vi "Register.vi"(6 "picture":refnum<vi>) -> (0 "error out":errorcluster)   [LabVIEW 2013]
uses:
  ROS/Code/SubVIs/BaxterSide.ctl
  ROS/Code/Console/Servers/ServerSubs/(nist) Arm Globals.vi
  <vilib>/Utility/config.llb/Read Key (String).vi
  <vilib>/Utility/config.llb/Read Key (Double).vi
  <vilib>/Utility/config.llb/Write Key (String).vi
  <vilib>/Utility/config.llb/NI_LVConfig.lvlib
panel:
  in  "Side":T1=enum."right"
  in  "Object":string
  in  "Tab Control":T2(tab)=enum."Calibration Table"
  out "picture 2":picture
  out "Progress":T3
  out "Table":dbl[][](array[numeric]) caption="FL\nFR\nNL\nNR" format="%.1f"
  # "Basic Commands are:\n   Convert   - convert offset to joints\n   Current   - current joint and offset\n   Register  - determine position\n   Save      - save calibration data\n   Load      - load calibration data\n   Reference - give reference joint position"
  # "Position gripper over center before starting"
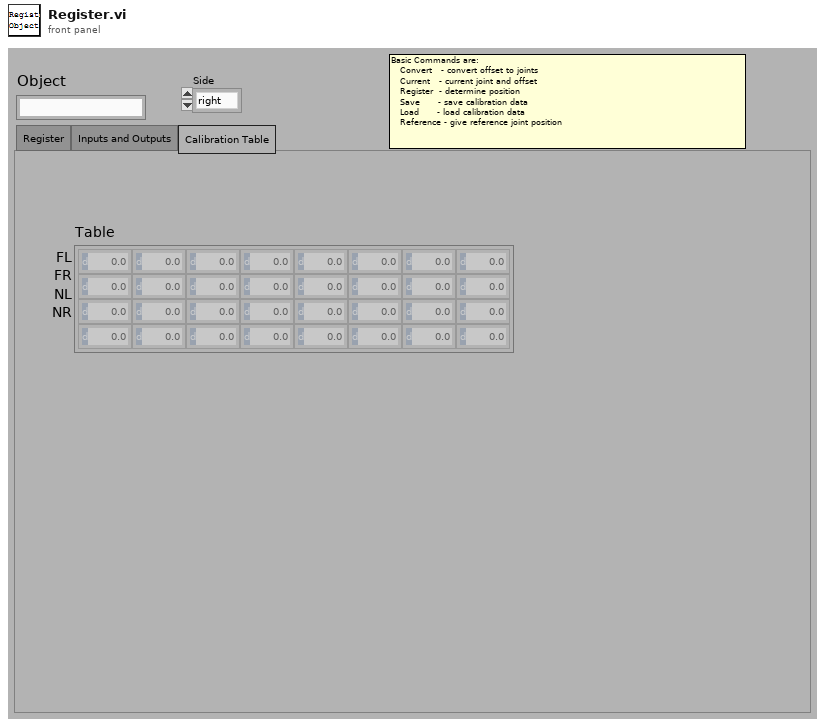
[diagram p1: front panel]
types:
  T1 = typedef "BaxterSide.ctl" = enum16{"left", "right"}
  T2 = enum32{"Register", "Inputs and Outputs", "Calibration Table"}
  T3 = cluster{"FL":bool, "FR":bool, "NL":bool, "NR":bool}
  T4 = cluster{"X":dbl, "Y":dbl, "Z":dbl, "O":dbl, "A":dbl, "T":dbl}
  T5 = typedef "NI_LVConfig.lvlib/Config Data RefNum.ctl" = refnum<k1>
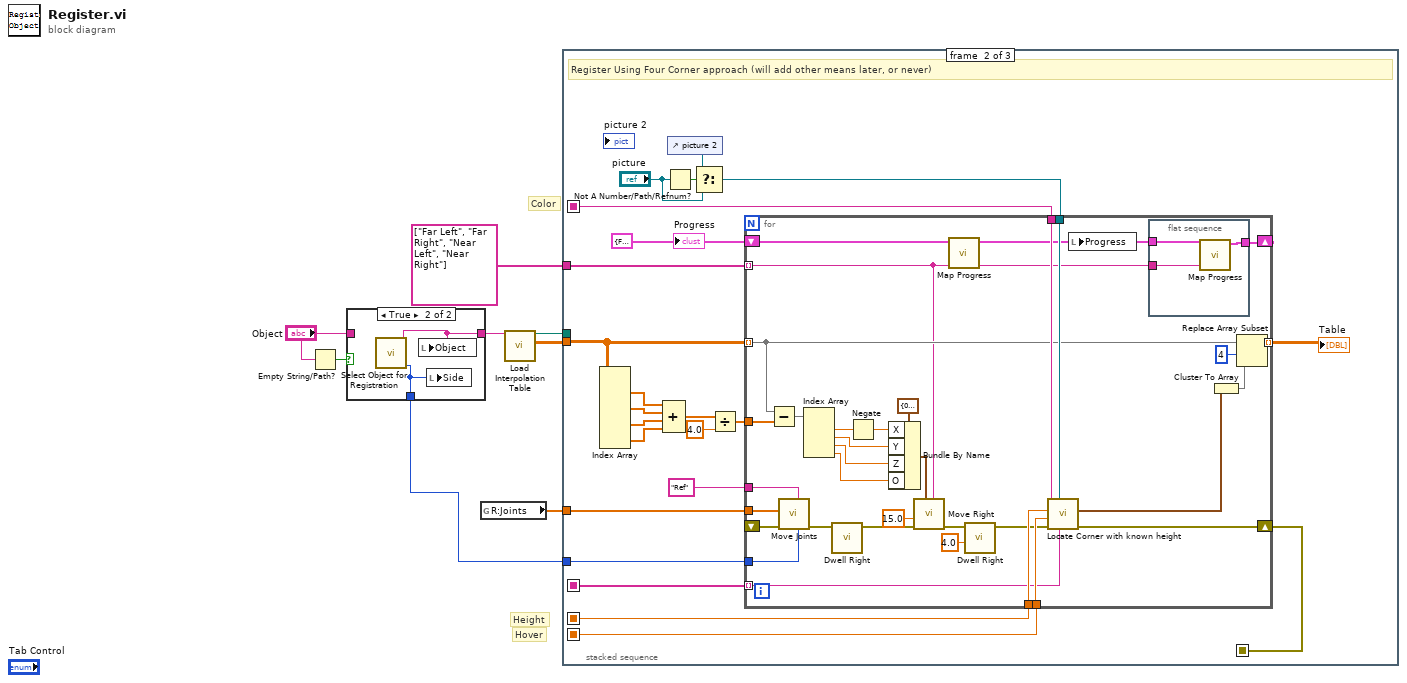
[diagram p0: block diagram]
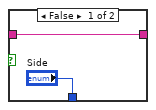
[diagram p2: hidden frame]
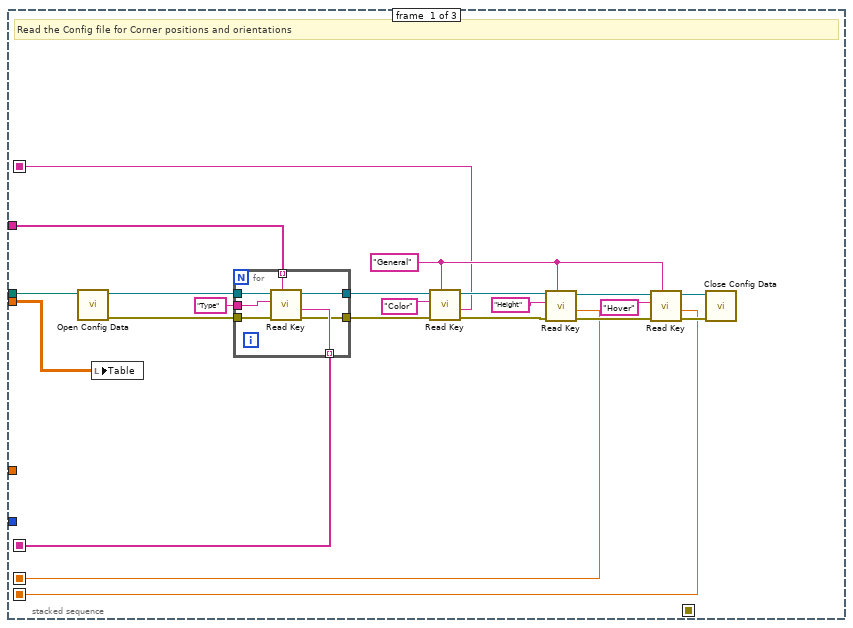
[diagram p3: hidden frame]
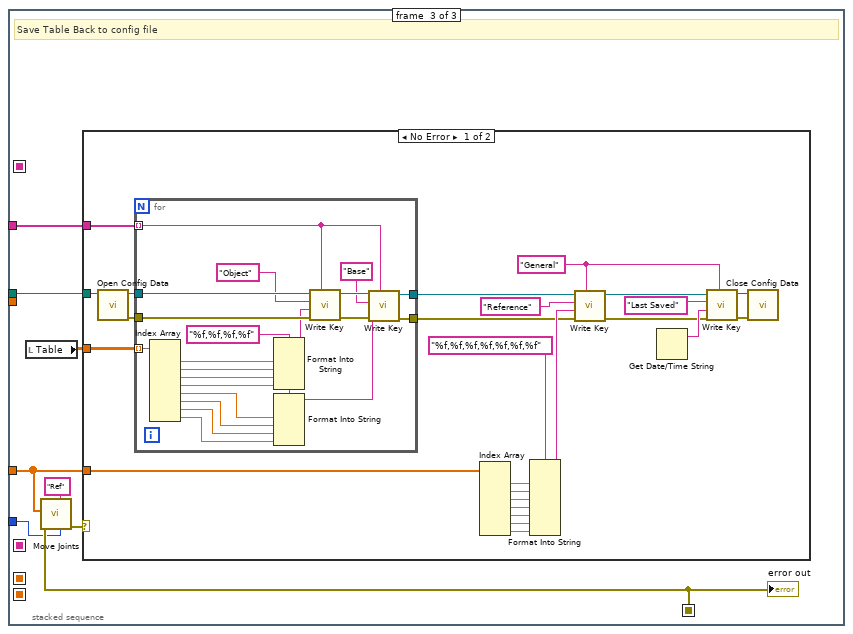
[diagram p4: hidden frame]
diagram:
  # "Color"
  # "Hover"
  # "Height"
  n1 = Empty String/Path?(string/path="Object") -> (empty?=w6:bool)
  n2 = case shown="True" w6 {
    tunnel: "Object" -> [w9 _]
    tunnel: ["Side" w11] -> w4
    tunnel: [w9 w12] -> w1
    frame False {
    }
    frame True {
      n3 = call "Select Object for Registration.vi"() -> ("Side"=w11:T1, "Object"=w12:string)  [unwired: 9 in, 1 out]
      n4 = local write "Object"(w12) -> ()
      n5 = local write "Side"(w11) -> ()
    }
  }
  n6 = global read "(nist) Arm Globals.vi" "R:Joints"() -> (w8:dbl[])
  n7 = call "Load Interpolation Table.vi"("Object Name"=w1) -> ("Table"=w3:dbl[][], "File"=w2:path)  [unwired: 7 in, 2 out]
  n8 = stacked-sequence {
    seq-local: [w15 _ _] -> [_ w54 _]
    seq-local: [w26 _ _] -> [_ w56 _]
    seq-local: [w27 _ _] -> [_ w55 _]
    seq-local: [w21 _ _] -> [_ w53 _]
    seq-local: [_ w44 _] -> [_ _ w105]
    tunnel: w8 -> [_ w42 w106]
    tunnel: w4 -> [_ w57 w102]
    tunnel: w2 -> [w34 _ w109]
    tunnel: w3 -> [w20 w52 _]
    tunnel: string[] ["Far Left", "Far Right", "Near Left", "Near Right"] -> [w19 w47 w108]
    frame #0 {
      w22 = "General" ("section")
      # "Read the Config file for Corner positions and orientations"
      n9 = call <vilib>:"Open Config Data.vi"("configuration file path"=w34) -> ("error out"=w17:errorcluster, "refnum"=w18:T5)  [unwired: 8 in, 1 out]
      n10 = local write "Table"(w20) -> ()
      n11 = for {
        tunnel: w19 -> [w41] mode=indexing
        tunnel: w18 -> [w40]
        tunnel: w17 -> [w39]
        tunnel: "Type" ("key") -> [w38]
        tunnel: [w37] -> w15 mode=indexing
        tunnel: [w36] -> w13
        tunnel: [w35] -> w14
        n12 = call-poly <vilib>:"Read Key.vi"("section"=w41, "error in (no error)"=w39, "key"=w38, "refnum"=w40) -> ("error out"=w36:errorcluster, "value"=w37:string, "refnum out"=w35:T5)  [unwired: 4 in, 1 out]
      }
      n13 = call-poly <vilib>:"Read Key.vi"("section"=w22, "error in (no error)"=w13, "key"="Color", "refnum"=w14) -> ("error out"=w23:errorcluster, "value"=w21:string, "refnum out"=w24:T5)  [unwired: 4 in, 1 out]
      n14 = call-poly <vilib>:"Read Key.vi"("section"=w22, "error in (no error)"=w23, "key"="Height", "refnum"=w24) -> ("error out"=w28:errorcluster, "value"=w26:dbl, "refnum out"=w31:T5)  [unwired: 4 in, 1 out]
      n15 = call-poly <vilib>:"Read Key.vi"("section"=w22, "error in (no error)"=w28, "key"="Hover", "refnum"=w31) -> ("error out"=w29:errorcluster, "value"=w27:dbl, "refnum out"=w30:T5)  [unwired: 4 in, 1 out]
      n16 = call <vilib>:"Close Config Data.vi"("error in (no error)"=w29, "refnum"=w30) -> ()  [unwired: 8 in, 2 out]
    }
    frame #1 {
      w46 = T3 {"FL"=FALSE, "FR"=FALSE, "NL"=FALSE, "NR"=FALSE} ("Progress")
      # "Register Using Four Corner approach (will add other means later, or never)"
      n17 = Index Array(array=w52) -> (element #1=w51:dbl[], element #2=w50:dbl[], element #3=w49:dbl[], element #4=w48:dbl[])  [unwired: 8 in]
      n18 = Compound Arithmetic op=ADD(w51, w50, w49, w48) -> (w62:dbl[])
      n19 = Not A Number/Path/Refnum?(number/path/refnum="picture") -> (NaN/Path/Refnum?=w59:bool)
      n20 = control-ref of="picture 2"() -> (w61:refnum<vi>)
      n21 = Select(t=w61, s=w59, f="picture") -> (s? t:f=w58:refnum<vi>)
      n22 = Divide(x=w62, y=4.0) -> (x/y=w64:dbl[])
      n23 = for {
        tunnel: w53 -> [w98]
        tunnel: w58 -> [w97]
        tunnel: w57 -> [w96]
        tunnel: w42 -> [w95]
        tunnel: w64 -> [w94]
        tunnel: w55 -> [w89]
        tunnel: w56 -> [w88]
        tunnel: [w75] -> w43 mode=indexing
        tunnel: w52 -> [w78] mode=indexing
        tunnel: w54 -> [w83] mode=indexing
        shift-right: [w81] -> w44
        shift-left: _ -> [w82]
        shift-right: [w73] -> _
        shift-left: w46 -> [w80]
        tunnel: w47 -> [w72] mode=indexing
        tunnel: "Ref" ("Label") -> [w79]
        n24 = Subtract(x=w78, y=w94) -> (x-y=w91:dbl[])
        n25 = call "Move Joints.vi"("Side"=w96, "Label"=w79, "error in"=w82, "Goal"=w95) -> ("error out"=w68:errorcluster)  [unwired: 6 in, 1 out]
        n26 = Index Array(array=w91) -> (element #1=w93:dbl, element #2=w87:dbl, element #3=w86:dbl, element #4=w85:dbl)  [unwired: 4 in]
        n27 = call "Dwell Right.vi"("error in"=w68) -> ("error out"=w67:errorcluster)  [unwired: 10 in]
        n28 = Negate(x=w93) -> (-x=w90:dbl)
        n29 = Bundle By Name(cluster=T4 {"X"=0.0, "Y"=0.0, "Z"=0.0, "O"=0.0, "A"=0.0, "T"=0.0} ("Goal Axes"), "X"=w90, "Y"=w87, "Z"=w86, "O"=w85) -> (w71:T4)
        n30 = call "Move Right.vi"("Label"=w72, "Goal"=w71, "error in"=w67, "Speed"=15.0) -> ("error out"=w70:errorcluster)  [unwired: 3 in, 4 out]
        n31 = call "Map Progress.vi"("Corner"=w72, "In"=w80) -> ("Out"=w74:T3)  [unwired: 9 in]
        n32 = call "Dwell Right.vi"("Wait Time"=4.0 ("wait time"), "error in"=w70) -> ("error out"=w69:errorcluster)  [unwired: 9 in]
        n33 = call "Locate Corner with known height.vi"("Corner Type"=w83, "picture"=w97, "error in"=w69, "Hover"=w89, "Height"=w88, "color"=w98) -> ("error out"=w81:errorcluster, "Robot Pose"=w84:cluster{"X":dbl, "Y":dbl, "Z":dbl, "A":dbl})  [unwired: 3 in, 1 out]
        n34 = local write "Progress"(w74) -> ()
        n35 = flat-sequence {
          tunnel: w74 -> [w101]
          tunnel: [w100] -> w73
          tunnel: w72 -> [w99]
          frame #0 {
            n36 = call "Map Progress.vi"("Corner"=w99, "In"=w101) -> ("Out"=w100:T3)  [unwired: 9 in]
          }
        }
        n37 = Cluster To Array(cluster=w84) -> (array=w76:dbl[])
        n38 = Replace Array Subset(array=w78, new element=w76, index=4) -> (w75:dbl[])
      }
      "Table" <- w43
      "Progress" <- w46
    }
    frame #2 {
      # "Save Table Back to config file"
      n39 = local read "Table"() -> (w107:dbl[][])
      n40 = call "Move Joints.vi"("Side"=w102, "Label"="Ref", "error in"=w105, "Goal"=w106) -> ("error out"=w104:errorcluster)  [unwired: 6 in, 1 out]
      n41 = case shown="No Error" w104 {
        tunnel: w109 -> [w132 _]
        tunnel: w108 -> [w114 _]
        tunnel: w106 -> [w111 _]
        tunnel: w107 -> [w110 _]
        frame No Error {
          w129 = "General" ("section")
          n42 = call <vilib>:"Open Config Data.vi"("configuration file path"=w132) -> ("error out"=w134:errorcluster, "refnum"=w133:T5)  [unwired: 8 in, 1 out]
          n43 = for {
            tunnel: w134 -> [w155]
            tunnel: w133 -> [w154]
            tunnel: w114 -> [w137] mode=indexing
            tunnel: w110 -> [w146] mode=indexing
            tunnel: [w136] -> w113
            tunnel: [w135] -> w112
            w148 = "%f,%f,%f,%f" ("format string")
            n44 = Index Array(array=w146) -> (element #1=w145:dbl, element #2=w144:dbl, element #3=w143:dbl, element #4=w142:dbl, element #5=w141:dbl, element #6=w140:dbl, element #7=w139:dbl, element #8=w138:dbl)  [unwired: 8 in]
            n45 = Format Into String(format string=w148, w145, w144, w143, w142) -> (resulting string=w152:string)  [unwired: 2 in, 1 out]
            n46 = Format Into String(format string=w148, w141, w140, w139, w138) -> (resulting string=w147:string)  [unwired: 2 in, 1 out]
            n47 = call-poly <vilib>:"Write Key.vi"("section"=w137, "error in (no error)"=w155, "value"=w152, "key"="Object", "refnum"=w154) -> ("error out"=w150:errorcluster, "refnum out"=w151:T5)  [unwired: 4 in, 1 out]
            n48 = call-poly <vilib>:"Write Key.vi"("section"=w137, "error in (no error)"=w150, "value"=w147, "key"="Base", "refnum"=w151) -> ("error out"=w135:errorcluster, "refnum out"=w136:T5)  [unwired: 4 in, 1 out]
          }
          n49 = Index Array(array=w111) -> (element #1=w119:dbl, element #2=w120:dbl, element #3=w121:dbl, element #4=w122:dbl, element #5=w123:dbl, element #6=w124:dbl, element #7=w125:dbl)  [unwired: 7 in]
          n50 = Format Into String(format string="%f,%f,%f,%f,%f,%f,%f", w119, w120, w121, w122, w123, w124, w125) -> (resulting string=w126:string)  [unwired: 2 in, 1 out]
          n51 = call-poly <vilib>:"Write Key.vi"("section"=w129, "error in (no error)"=w112, "value"=w126, "key"="Reference", "refnum"=w113) -> ("error out"=w128:errorcluster, "refnum out"=w127:T5)  [unwired: 4 in, 1 out]
          n52 = Get Date/Time String() -> (date string=w130:string)  [unwired: 3 in, 1 out]
          n53 = call-poly <vilib>:"Write Key.vi"("section"=w129, "error in (no error)"=w128, "value"=w130, "key"="Last Saved", "refnum"=w127) -> ("error out"=w115:errorcluster, "refnum out"=w116:T5)  [unwired: 4 in, 1 out]
          n54 = call <vilib>:"Close Config Data.vi"("error in (no error)"=w115, "refnum"=w116) -> ()  [unwired: 8 in, 2 out]
        }
        frame Error {
        }
      }
      "error out" <- w105
    }
  }
